vi "GetProperties.vi"(8 "error in":errorcluster, 11 "Pane in":refnum<class "Pane.lvclass">) -> (0 "error out":errorcluster, 3 "Pane out":refnum<class "Pane.lvclass">)   [LabVIEW 2014, in "Raspberry Pi Compatible Compiler for LabVIEW.lvlib" / "Pane.lvclass"]
uses:
  Pane.lvclass
  Pane.lvclass/Pane.ctl
  GObject/GObject.lvclass
  Text/Text.lvclass
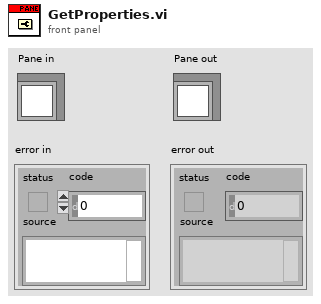
[diagram p1: front panel]
types:
  T1 = typedef "imagedata.ctl" = cluster{"image type":i32, "image depth":i32, "image":u8[], "mask":u8[], "colors":u32[], "Rectangle":cluster{"left":i16, "top":i16, "right":i16, "bottom":i16}}
  T2 = enum16{"Always On", "Always Off", "Off While Running"}
  T3 = typedef "LVPointTypeDef.ctl" = cluster{"Horizontal":i16, "Vertical":i16}
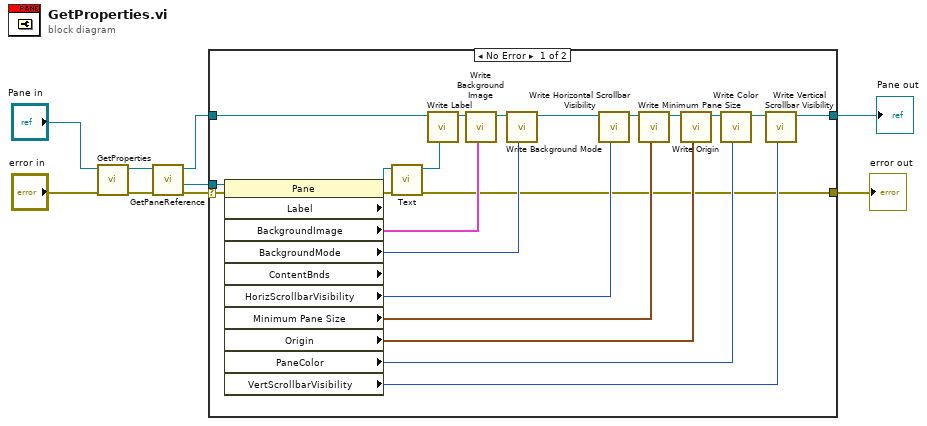
[diagram p0: block diagram]
diagram:
  n1 = call-parent "GetProperties.vi"("error in"="error in", "GObject in"="Pane in") -> ("error out"=w6:errorcluster, "GObject out"=w7:refnum<class "Pane.lvclass">)  [unwired: 8 in]
  n2 = call "GetPaneReference.vi"("error in"=w6, "Pane in"=w7) -> ("error out"=w5:errorcluster, "pane reference"=w4:refnum<vi>, "Pane out"=w3:refnum<class "Pane.lvclass">)  [unwired: 7 in]
  n3 = case shown="No Error" w5 {
    selector: w5 -> [w31 w32]
    tunnel: w4 -> [w30 _]
    tunnel: w3 -> [w12 w33]
    tunnel: [w11 w32] -> w2
    tunnel: [w10 w33] -> w1
    frame No Error {
      n4 = property class="Pane" props=["Label", "BackgroundImage", "BackgroundMode", "ContentBnds", "HorizScrollbarVisibility", "Minimum Pane Size", "Origin", "PaneColor", "VertScrollbarVisibility"](reference=w30, error in=w31) -> (error out=w16:errorcluster, "Label"=w15:refnum<vi>, "BackgroundImage"=w29:T1, "BackgroundMode"=w27:enum16{"Stretch", "Center", "Tile"}, "HorizScrollbarVisibility"=w26:T2, "Minimum Pane Size"=w23:T3, "Origin"=w21:T3, "PaneColor"=w19:u32, "VertScrollbarVisibility"=w17:T2)  [unwired: 2 out]
      n5 = call "Text.vi"("error in"=w16, "Gen Refnum"=w15) -> ("error out"=w11:errorcluster, "Text out"=w13:refnum<class "Text.lvclass">)  [unwired: 8 in]
      n6 = call "Write Label.vi"("Label"=w13, "Pane in"=w12) -> ("Pane out"=w14:refnum<class "Pane.lvclass">)  [unwired: 7 in]
      n7 = call "Write Background Image.vi"("image data"=w29, "Pane in"=w14) -> ("Pane out"=w28:refnum<class "Pane.lvclass">)  [unwired: 7 in]
      n8 = call "Write Background Mode.vi"("Background Mode"=w27, "Pane in"=w28) -> ("Pane out"=w25:refnum<class "Pane.lvclass">)  [unwired: 7 in]
      n9 = call "Write Horizontal Scrollbar Visibility.vi"("Horizontal Scrollbar Visibility"=w26, "Pane in"=w25) -> ("Pane out"=w24:refnum<class "Pane.lvclass">)  [unwired: 7 in]
      n10 = call "Write Minimum Pane Size.vi"("Minimum Pane Size"=w23, "Pane in"=w24) -> ("Pane out"=w22:refnum<class "Pane.lvclass">)  [unwired: 7 in]
      n11 = call "Write Origin.vi"("Origin"=w21, "Pane in"=w22) -> ("Pane out"=w20:refnum<class "Pane.lvclass">)  [unwired: 7 in]
      n12 = call "Write Color.vi"("Color"=w19, "Pane in"=w20) -> ("Pane out"=w18:refnum<class "Pane.lvclass">)  [unwired: 7 in]
      n13 = call "Write Vertical Scrollbar Visibility.vi"("Vertical Scrollbar Visibility"=w17, "Pane in"=w18) -> ("Pane out"=w10:refnum<class "Pane.lvclass">)  [unwired: 7 in]
    }
    frame Error {
    }
  }
  "error out" <- w2
  "Pane out" <- w1
